vi "Apply Setpoints.vi"(8 "error in":errorcluster, 11 "6032A in":refnum<class "6032A.lvclass">) -> (0 "error out":errorcluster, 3 "6032A out":refnum<class "6032A.lvclass">)   [LabVIEW 2019, in "6032A.lvlib" / "6032A.lvclass"]
uses:
  Library/6032A.lvclass
  C:/Users/Public/Documents/Development/builds/Instruments/PowerSupply.lvlibp/Library/PowerSupply.lvclass
  Library/6032A.lvclass/6032A.ctl
  <instrlib>/Agilent 6XXX Series/Agilent 6XXX Series.lvlib
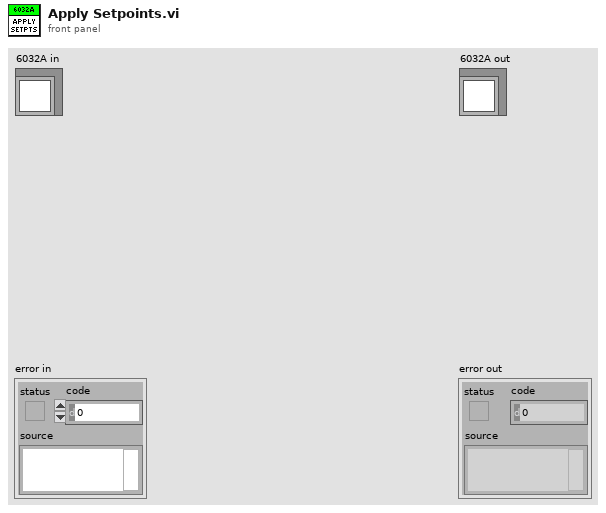
[diagram p1: front panel]
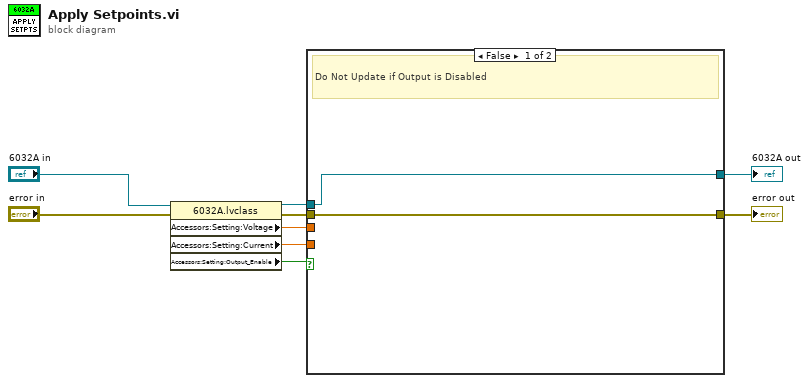
[diagram p0: block diagram]
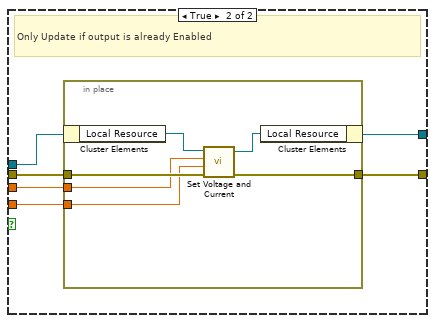
[diagram p2: hidden frame]
diagram:
  n1 = property class="6032A.lvclass"(reference="6032A in", error in="error in") -> (reference out=w6:refnum<class "6032A.lvclass">, error out=w5:errorcluster, "Accessors:Setting:Voltage"=w3:dbl, "Accessors:Setting:Current"=w2:dbl, "Accessors:Setting:Output_Enable"=w1:bool)
  n2 = case shown="False" w1 {
    tunnel: [w11 w17] -> w9
    tunnel: w6 -> [w11 w16]
    tunnel: w5 -> [w10 w15]
    tunnel: [w10 w14] -> w4
    tunnel: w3 -> [_ w13]
    tunnel: w2 -> [_ w12]
    frame False {
      # "Do Not Update if Output is Disabled"
    }
    frame True {
      # "Only Update if output is already Enabled"
      n3 = in-place {
        in-place-border: w15 -> [w21]
        in-place-border: [w20] -> w14
        in-place-border: w13 -> [w19]
        in-place-border: w12 -> [w18]
        n4 = in-place-cluster #1(w16) -> ("Local Resource"=w23:refnum<visa-resource-name>)
        n5 = call <instrlib>:"Set Voltage and Current.vi"("error in (no error)"=w21, "current (0 A)"=w18, "voltage (0 V)"=w19, "VISA resource name"=w23) -> ("error out"=w20:errorcluster, "VISA resource name out"=w22:refnum<visa-resource-name>)  [unwired: 6 in]
        n6 = in-place-cluster #1("Local Resource"=w22) -> (w17:refnum<class "6032A.lvclass">)
      }
    }
  }
  "error out" <- w4
  "6032A out" <- w9
